vi "_emi_Close Loop Single.vi"(5 "Loop ID in":u16, 9 "error in (no error)":errorcluster) -> (10 "error out":errorcluster)   [LabVIEW 2010]
doc: "Destroy the Loop, should be performed after the outer loop exists in prepreation of program close.\n\nExecutes as normal on error"
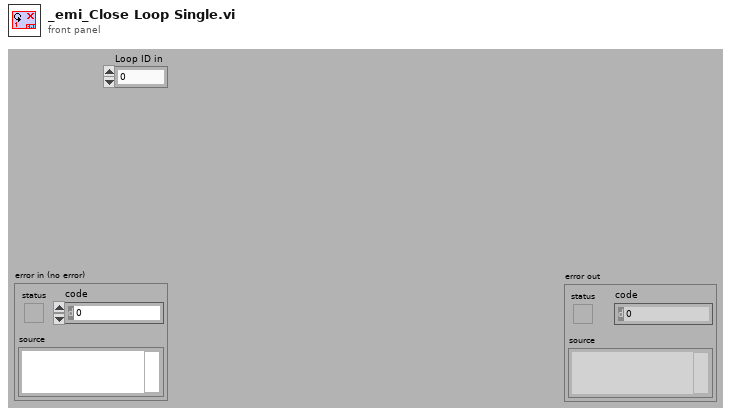
[diagram p1: front panel]
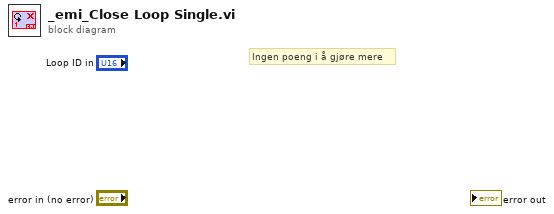
[diagram p0: block diagram]
diagram:
  # "Ingen poeng i å gjøre mere"
